vi "CreateMapImp.vi"(8 "error in (no error)":errorcluster, 11 "Map in":refnum<class "ObjectMap.lvclass">) -> (0 "error out":errorcluster, 3 "Map out":refnum<class "ObjectMap.lvclass">)   [LabVIEW 2013, in "LapDog.Collections.v_.Maps.lvlib" / "ObjectMap.lvclass"]
doc: "This method invokes the Map Implementation's \"Create\" method, which ensures implementations will work when end users connect implementation class contants to the Map.Create method.\n\nMap subclasses should call this method in their own Create methods."
uses:
  ObjectMap.lvclass
  MapImp/MapImp.lvclass
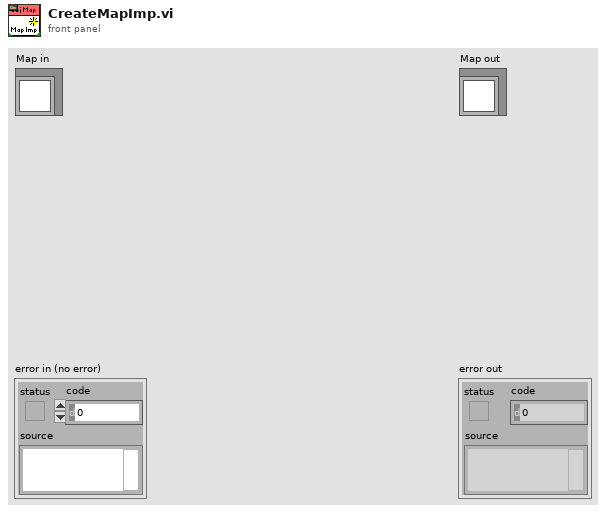
[diagram p1: front panel]
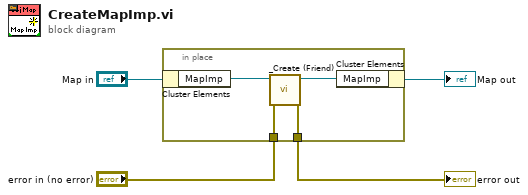
[diagram p0: block diagram]
diagram:
  n1 = in-place {
    in-place-border: "error in (no error)" -> [w6]
    in-place-border: [w5] -> w1
    n2 = in-place-cluster #1("Map in") -> ("MapImp"=w8:refnum<class "MapImp.lvclass">)
    n3 = call "_Create (Friend).vi"("error in (no error)"=w6, "MapImp in"=w8) -> ("error out"=w5:errorcluster, "MapImp out"=w7:refnum<class "MapImp.lvclass">)  [unwired: 8 in]
    n4 = in-place-cluster #1("MapImp"=w7) -> (→"Map out":refnum<class "ObjectMap.lvclass">)
  }
  "error out" <- w1
